vi "AddColData.vi"(8 "エラー入力（エラーなし）":errorcluster, 9 "名称":string, 10 "配列":dbl[](array[numeric]), 11 "Table入力":refnum<vi>) -> (0 "エラー出力":errorcluster)   [LabVIEW 2014]
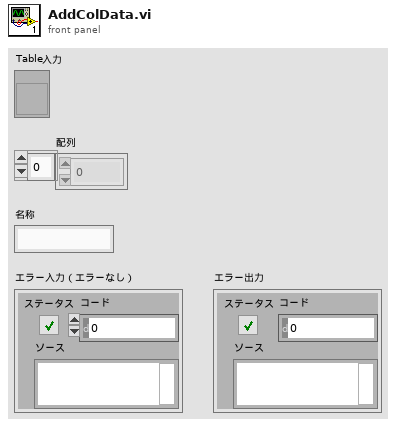
[diagram p1: front panel]
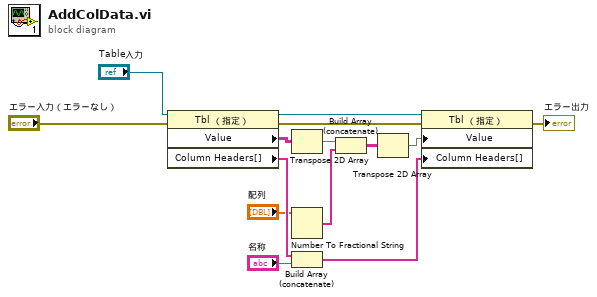
[diagram p0: block diagram]
diagram:
  n1 = property class="Tbl （指定）"(reference="Table入力", error in="エラー入力（エラーなし）") -> (reference out=w10:refnum<vi>, error out=w14:errorcluster, "Value"=w12:string[][], "Column Headers[]"=w11:string[])
  n2 = Transpose 2D Array(2D array=w12) -> (transposed array=w8:string[][])
  n3 = Number To Fractional String(number="配列") -> (F-format string=w3:string[])  [unwired: 3 in]
  n4 = Build Array (concatenate)(w11, "名称") -> (w6:string[])
  n5 = Build Array (concatenate)(w8, w3) -> (w1:string[][])
  n6 = Transpose 2D Array(2D array=w1) -> (transposed array=w5:string[][])
  n7 = property class="Tbl （指定）"(reference=w10, error in=w14, "Value"=w5, "Column Headers[]"=w6) -> (error out=→"エラー出力":errorcluster)  [unwired: 1 out]
